vi "CANStrView.vi"(6 "StrInit":string, 7 "ID":string, 8 "error in":errorcluster caption="错误输入", 9 "CANStrView":refnum<vi>, 10 "DataRec":string, 11 "DataTrans":string) -> (0 "error out":errorcluster caption="错误输出", 3 "连接显示":string)   [LabVIEW 2013]
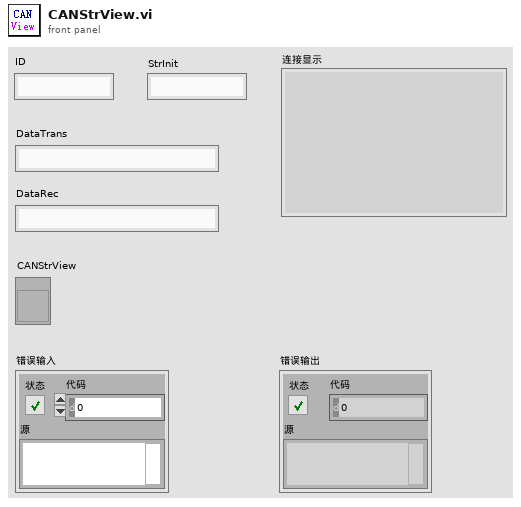
[diagram p1: front panel]
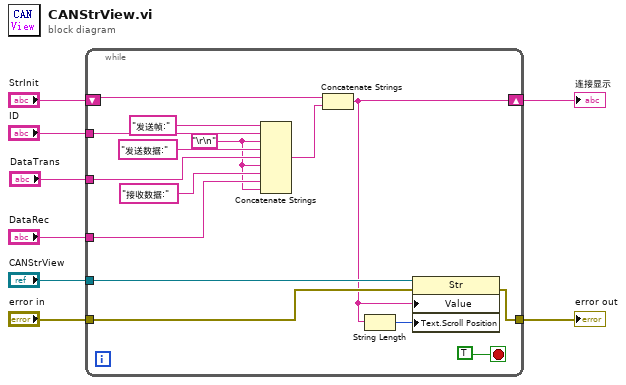
[diagram p0: block diagram]
diagram:
  n1 = while {
    tunnel: "ID" -> [w22]
    tunnel: "DataTrans" -> [w20]
    tunnel: "DataRec" -> [w18]
    tunnel: "CANStrView" -> [w16]
    tunnel: "error in" -> [w15]
    tunnel: [w14] -> w3
    shift-right: [w9] -> w2
    shift-left: "StrInit" -> [w12]
    stop <- TRUE stop-if-true
    w17 = "\r\n"
    n2 = Concatenate Strings("发送帧:", w22, w17, "发送数据:", w20, w17, "接收数据:", w18, w17) -> (w11:string)
    n3 = Concatenate Strings(w12, w11) -> (w9:string)
    n4 = String Length(string=w9) -> (length=w10:i32)
    n5 = property class="Str"(reference=w16, error in=w15, "Value"=w9, "Text.Scroll Position"=w10) -> (error out=w14:errorcluster)  [unwired: 1 out]
  }
  "error out" <- w3
  "连接显示" <- w2
